vi "WPI_CameraGet Image Notifier Internal.vi"(8 "error in (no error)":errorcluster, 11 "Camera Address":string) -> (0 "error out":errorcluster, 3 "Image Notifier":refnum<notifier>)   [LabVIEW 2017]
doc: "This software is licensed. Open the labview\\readme\\WPI Robotics Library Open Source License.txt file for more information."
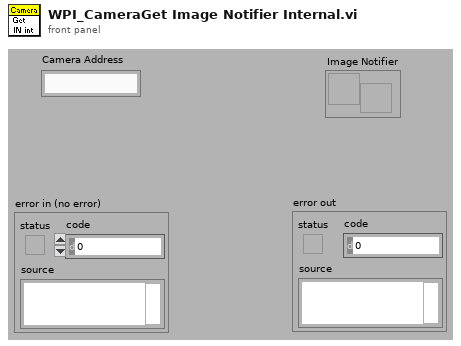
[diagram p1: front panel]
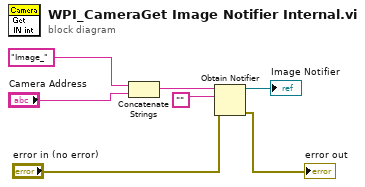
[diagram p0: block diagram]
diagram:
  n1 = Concatenate Strings("Image_" ("format string"), "Camera Address") -> (w3:string)
  n2 = Obtain Notifier(name (unnamed)=w3, notification data type="", error in (no error)="error in (no error)") -> (notifier out=→"Image Notifier":refnum<notifier>, error out=→"error out":errorcluster)  [unwired: 1 in, 1 out]
